vi "LDA_stats.vi"(0 "Eng Units":dbl[][](array[numeric]) format="%.2f", 1 "dimensions":enum16{"1D", "2D"}(ring)=enum."2D", 2 "Info Index":i32, 5 "Indicies":i32[](array[numeric]), 9 "Inst names":string[](array[string]), 11 "Shift in":dbl[](array[numeric]) format="%.2f", 12 "Block No":i32, 13 "Weighting":dbl[](array[numeric]) format="%.2f") -> (4 "Results file string array":string[](array[string]), 15 "Shift out":dbl[](array[numeric]) format="%.2f")   [LabVIEW 2010]
uses:
  Globals/Meas_global.vi
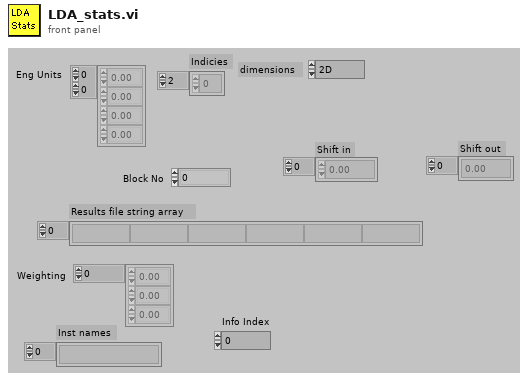
[diagram p1: front panel]
types:
  T1 = typedef "Velocity_cluster.ctl" = cluster{"Name":string, "U":dbl, "u^2":dbl, "u^3/(u^2)^(1.5)":dbl, "u^4/(u^2)^2 -3":dbl, "% u'/U":dbl, "Mean % Err":dbl, "u^4":dbl}
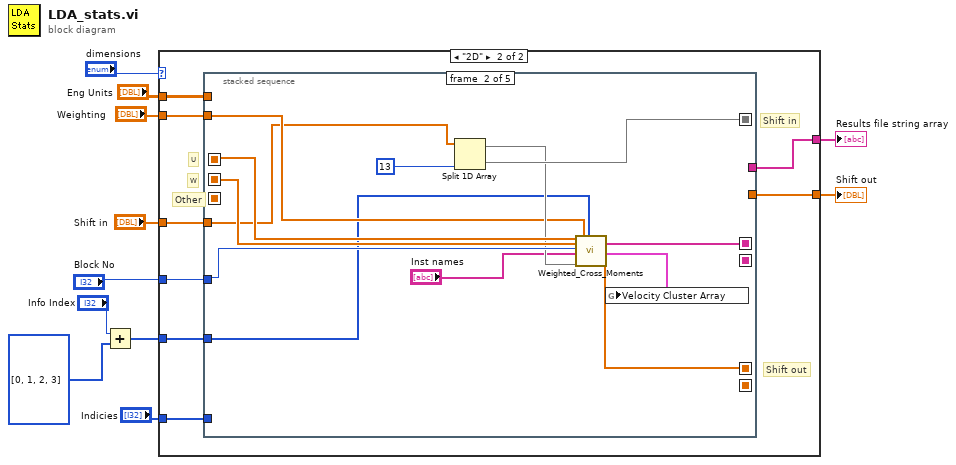
[diagram p0: block diagram]
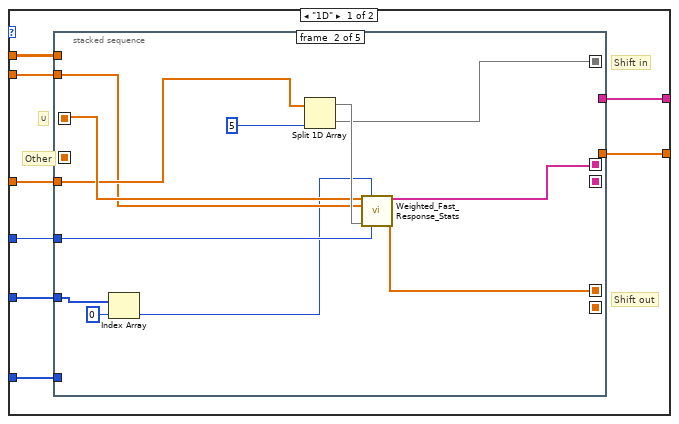
[diagram p2: hidden frame]
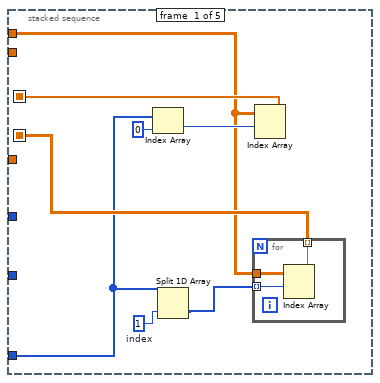
[diagram p3: hidden frame]
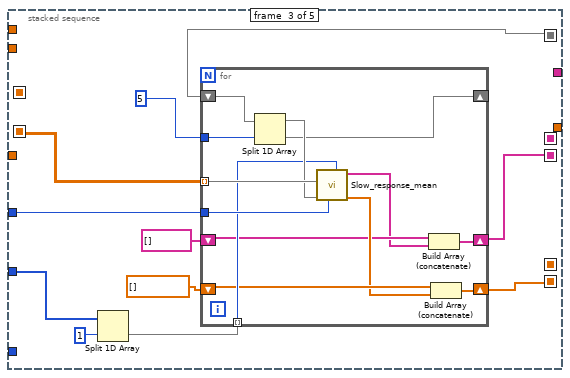
[diagram p4: hidden frame]
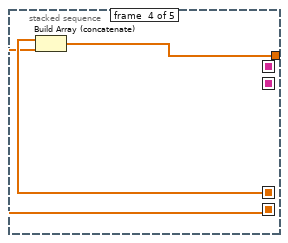
[diagram p5: hidden frame]
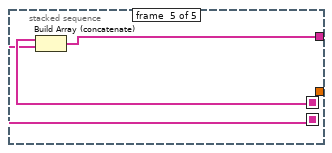
[diagram p6: hidden frame]
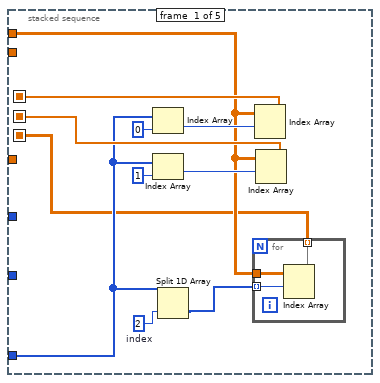
[diagram p7: hidden frame]
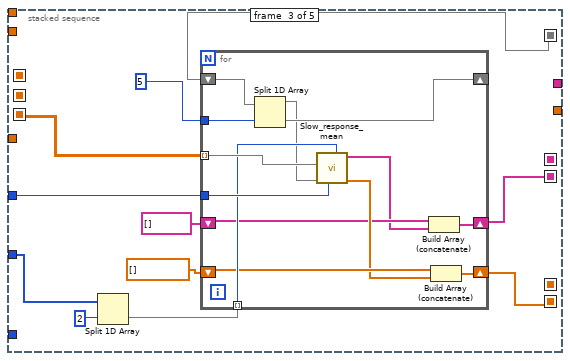
[diagram p8: hidden frame]
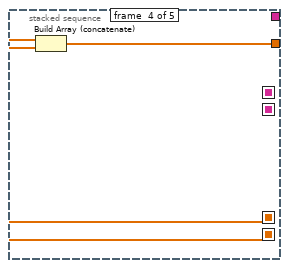
[diagram p9: hidden frame]
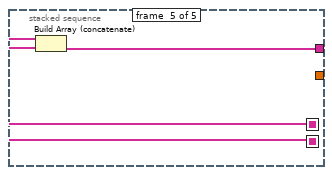
[diagram p10: hidden frame]
diagram:
  n1 = Add(x="Info Index", y=i32[] [0, 1, 2, 3] ("x+y")) -> (x+y=w2:i32[])
  n2 = case shown="\"2D\"" "dimensions" {
    tunnel: "Block No" -> [w19 w80]
    tunnel: [w18 w79] -> w10
    tunnel: "Eng Units" -> [w17 w78]
    tunnel: "Indicies" -> [w16 w77]
    tunnel: "Shift in" -> [w15 w76]
    tunnel: [w14 w75] -> w6
    tunnel: "Weighting" -> [w13 w74]
    tunnel: w2 -> [w12 w73]
    frame "1D" {
      # "U"
      # "Other"
      # "Shift in"
      # "Shift out"
      n3 = stacked-sequence {
        seq-local: [w25 _ _ _ _] -> [_ w36 _ _ _]
        seq-local: [w22 _ _ _ _] -> [_ _ w51 _ _]
        seq-local: [_ w40 _ _ _] -> [_ _ w46 _ _]
        seq-local: [_ w39 _ _ _] -> [_ _ _ w69 _]
        seq-local: [_ _ w44 _ _] -> [_ _ _ w68 _]
        seq-local: [_ w38 _ _ _] -> [_ _ _ _ w72]
        seq-local: [_ _ w45 _ _] -> [_ _ _ _ w71]
        tunnel: w19 -> [_ w37 w52 _ _]
        tunnel: [_ _ _ w67 _] -> w18
        tunnel: w17 -> [w21 _ _ _ _]
        tunnel: w16 -> [w20 _ _ _ _]
        tunnel: w15 -> [_ w35 _ _ _]
        tunnel: [_ _ _ _ w70] -> w14
        tunnel: w13 -> [_ w34 _ _ _]
        tunnel: w12 -> [_ w33 w43 _ _]
        frame #0 {
          w24 = 1  # index
          n4 = Index Array(array=w20, index=0) -> (element=w26:i32)
          n5 = Split 1D Array(array=w20, index=w24) -> (second subarray=w23:i32[])  [unwired: 1 out]
          n6 = for {
            tunnel: w21 -> [w30]
            tunnel: w23 -> [w29] mode=indexing
            tunnel: [w28] -> w22 mode=indexing
            n7 = Index Array(array=w30, index (row)=w29) -> (element=w28:dbl[])  [unwired: 1 in]
          }
          n8 = Index Array(array=w21, index (row)=w26) -> (element=w25:dbl[])  [unwired: 1 in]
        }
        frame #1 {
          n9 = Index Array(array=w33, index=0) -> (element=w31:i32)
          n10 = Split 1D Array(array=w35, index=5) -> (first subarray=w41:dbl[], second subarray=w40:dbl[])
          n11 = call "Weighted_Fast_Response_Stats.vi"("U"=w36, "Index"=w31, "Weighting"=w34, "Shift in"=w41, "Block No"=w37) -> ("Results file string array"=w38:string[], "Shift out"=w39:dbl[])  [unwired: 3 in, 6 out]
        }
        frame #2 {
          n12 = Split 1D Array(array=w43, index=1) -> (second subarray=w48:i32[])  [unwired: 1 out]
          n13 = for {
            tunnel: w51 -> [w66] mode=indexing
            tunnel: w52 -> [w64]
            tunnel: w48 -> [w63] mode=indexing
            tunnel: 5 -> [w62]
            shift-right: [w60] -> _
            shift-left: w46 -> [w61]
            shift-right: [w57] -> w44
            shift-left: dbl[] [] -> [w59]
            shift-right: [w55] -> w45
            shift-left: string[] [] -> [w56]
            n14 = Split 1D Array(array=w61, index=w62) -> (first subarray=w65:dbl[], second subarray=w60:dbl[])
            n15 = call "Slow_response_mean.vi"("Index"=w63, "Block No"=w64, "Shift in"=w65, "U"=w66) -> ("Shift out"=w58:dbl[], "Results file string array"=w54:string[])  [unwired: 4 out]
            n16 = Build Array (concatenate)(w56, w54) -> (w55:string[])
            n17 = Build Array (concatenate)(w59, w58) -> (w57:dbl[])
          }
        }
        frame #3 {
          n18 = Build Array (concatenate)(w69, w68) -> (w67:dbl[])
        }
        frame #4 {
          n19 = Build Array (concatenate)(w72, w71) -> (w70:string[])
        }
      }
    }
    frame "2D" {
      # "U"
      # "W"
      # "Other"
      # "Shift in"
      # "Shift out"
      n20 = stacked-sequence {
        seq-local: [w87 _ _ _ _] -> [_ w105 _ _ _]
        seq-local: [w86 _ _ _ _] -> [_ w104 _ _ _]
        seq-local: [w81 _ _ _ _] -> [_ _ w116 _ _]
        seq-local: [_ w102 _ _ _] -> [_ _ w115 _ _]
        seq-local: [_ w106 _ _ _] -> [_ _ _ w134 _]
        seq-local: [_ w98 _ _ _] -> [_ _ _ _ w137]
        seq-local: [_ _ w110 _ _] -> [_ _ _ _ w136]
        seq-local: [_ _ w113 _ _] -> [_ _ _ w133 _]
        tunnel: w80 -> [_ w103 w117 _ _]
        tunnel: [_ _ _ w132 _] -> w79
        tunnel: w78 -> [w83 _ _ _ _]
        tunnel: w77 -> [w84 _ _ _ _]
        tunnel: w76 -> [_ w99 _ _ _]
        tunnel: [_ _ _ _ w135] -> w75
        tunnel: w74 -> [_ w100 _ _ _]
        tunnel: w73 -> [_ w95 w108 _ _]
        frame #0 {
          w85 = 2  # index
          n21 = Index Array(array=w84, index=0) -> (element=w89:i32)
          n22 = Index Array(array=w84, index=1) -> (element=w88:i32)
          n23 = Split 1D Array(array=w84, index=w85) -> (second subarray=w82:i32[])  [unwired: 1 out]
          n24 = for {
            tunnel: w83 -> [w94]
            tunnel: w82 -> [w93] mode=indexing
            tunnel: [w92] -> w81 mode=indexing
            n25 = Index Array(array=w94, index (row)=w93) -> (element=w92:dbl[])  [unwired: 1 in]
          }
          n26 = Index Array(array=w83, index (row)=w89) -> (element=w87:dbl[])  [unwired: 1 in]
          n27 = Index Array(array=w83, index (row)=w88) -> (element=w86:dbl[])  [unwired: 1 in]
        }
        frame #1 {
          n28 = Split 1D Array(array=w99, index=13) -> (first subarray=w101:dbl[], second subarray=w102:dbl[])
          n29 = call "Weighted_Cross_Moments.vi"("U"=w105, "W"=w104, "Block No"=w103, "Inst names"="Inst names", "Shift in"=w101, "Weighting"=w100, "Indicies"=w95) -> ("All Results for file"=w98:string[], "Velocity Cluster Array Out"=w96:T1[], "Shift out"=w106:dbl[])  [unwired: 1 in, 9 out]
          n30 = global write "Meas_global.vi" "Velocity Cluster Array"(w96) -> ()
        }
        frame #2 {
          n31 = Split 1D Array(array=w108, index=2) -> (second subarray=w111:i32[])  [unwired: 1 out]
          n32 = for {
            tunnel: w116 -> [w131] mode=indexing
            tunnel: w117 -> [w130]
            tunnel: w111 -> [w129] mode=indexing
            tunnel: 5 -> [w128]
            shift-right: [w120] -> _
            shift-left: w115 -> [w127]
            shift-right: [w124] -> w113
            shift-left: dbl[] [] -> [w126]
            shift-right: [w122] -> w110
            shift-left: string[] [] -> [w123]
            n33 = Split 1D Array(array=w127, index=w128) -> (first subarray=w119:dbl[], second subarray=w120:dbl[])
            n34 = call "Slow_response_mean.vi"("Index"=w129, "Block No"=w130, "Shift in"=w119, "U"=w131) -> ("Shift out"=w125:dbl[], "Results file string array"=w121:string[])  [unwired: 4 out]
            n35 = Build Array (concatenate)(w123, w121) -> (w122:string[])
            n36 = Build Array (concatenate)(w126, w125) -> (w124:dbl[])
          }
        }
        frame #3 {
          n37 = Build Array (concatenate)(w134, w133) -> (w132:dbl[])
        }
        frame #4 {
          n38 = Build Array (concatenate)(w137, w136) -> (w135:string[])
        }
      }
    }
  }
  "Shift out" <- w10
  "Results file string array" <- w6
